vi "Header pkyk.vi"(8 "error in (no error)":errorcluster, 11 "New PKYK":T1) -> (0 "error out":errorcluster, 2 "MC No?":i32, 3 "PKYK":picture)   [LabVIEW 2020]
uses:
  MS SQL/MS_Global.vi
  Controls/Msg_Type.ctl
  Controls/Poka_Status.ctl
  Controls/PKYK_Status.ctl
  Controls/PKYK_Barcode_Status.ctl
  Controls/PKYK_qData.ctl
panel:
  # "Required\nResult"
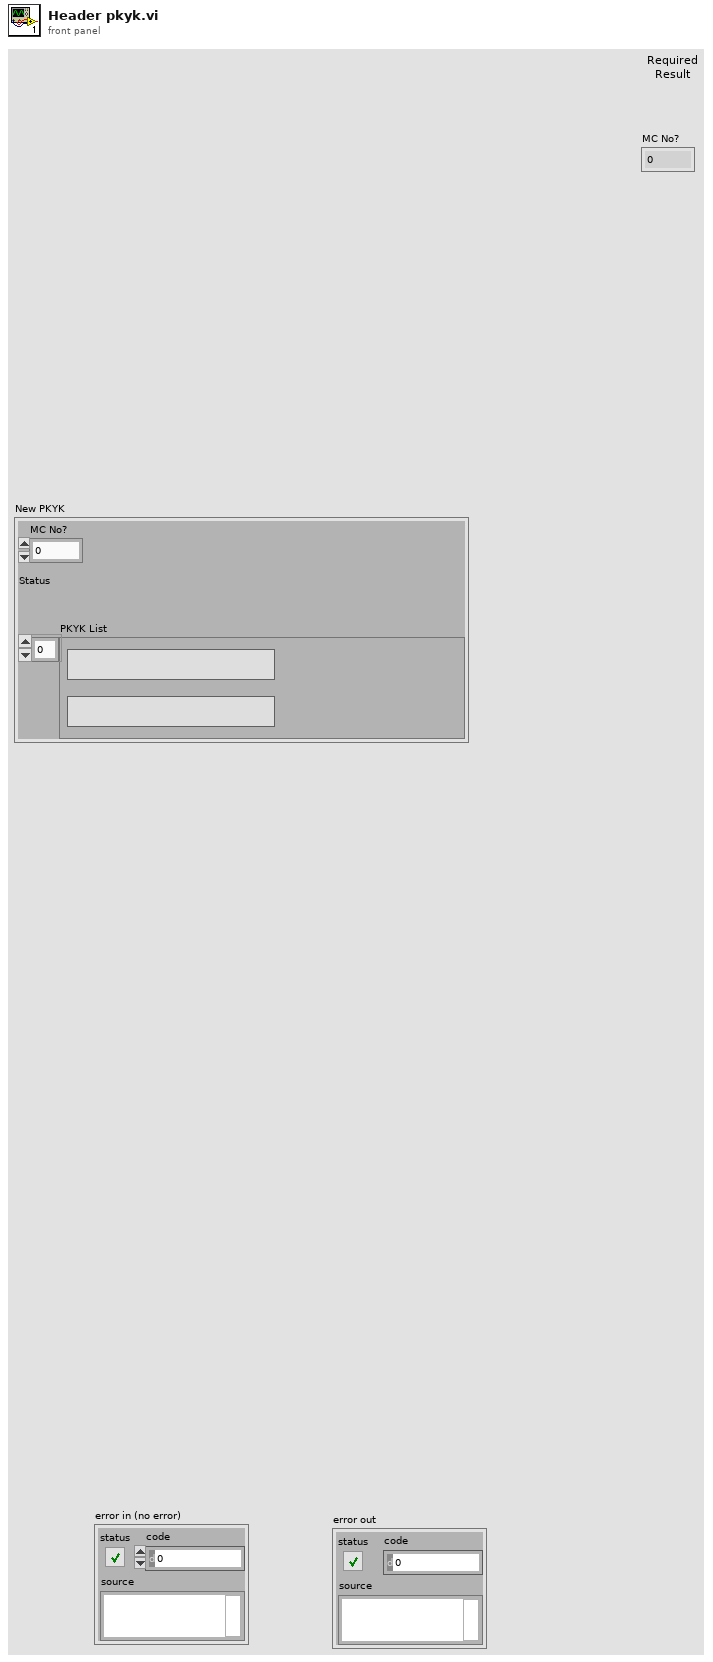
[diagram p1: front panel]
types:
  T1 = typedef "PKYK_qData.ctl" = cluster{"MC No?":i32, "Status":T2, "PKYK List":T3[]}
  T2 = typedef "Poka_Status.ctl" = u16
  T3 = typedef "PKYK_Barcode_Status.ctl" = cluster{"RFID Written Last":string, "Result":T4, "Exp. Result":T4}
  T4 = typedef "PKYK_Status.ctl" = u16
  T5 = typedef "Msg_Type.ctl" = enum16{"Normal", "Pass", "Fail", "Fault", "User", "Bypass", "Fail Save"}
  T6 = cluster{"left":i16, "top":i16, "right":i16, "bottom":i16}
  T7 = cluster{"Font Name:":string, "Size":i16, "Strikeout?":bool, "Italic?":bool, "Underline?":bool, "Outline?":bool, "Shadow?":bool, "Bold?":bool}
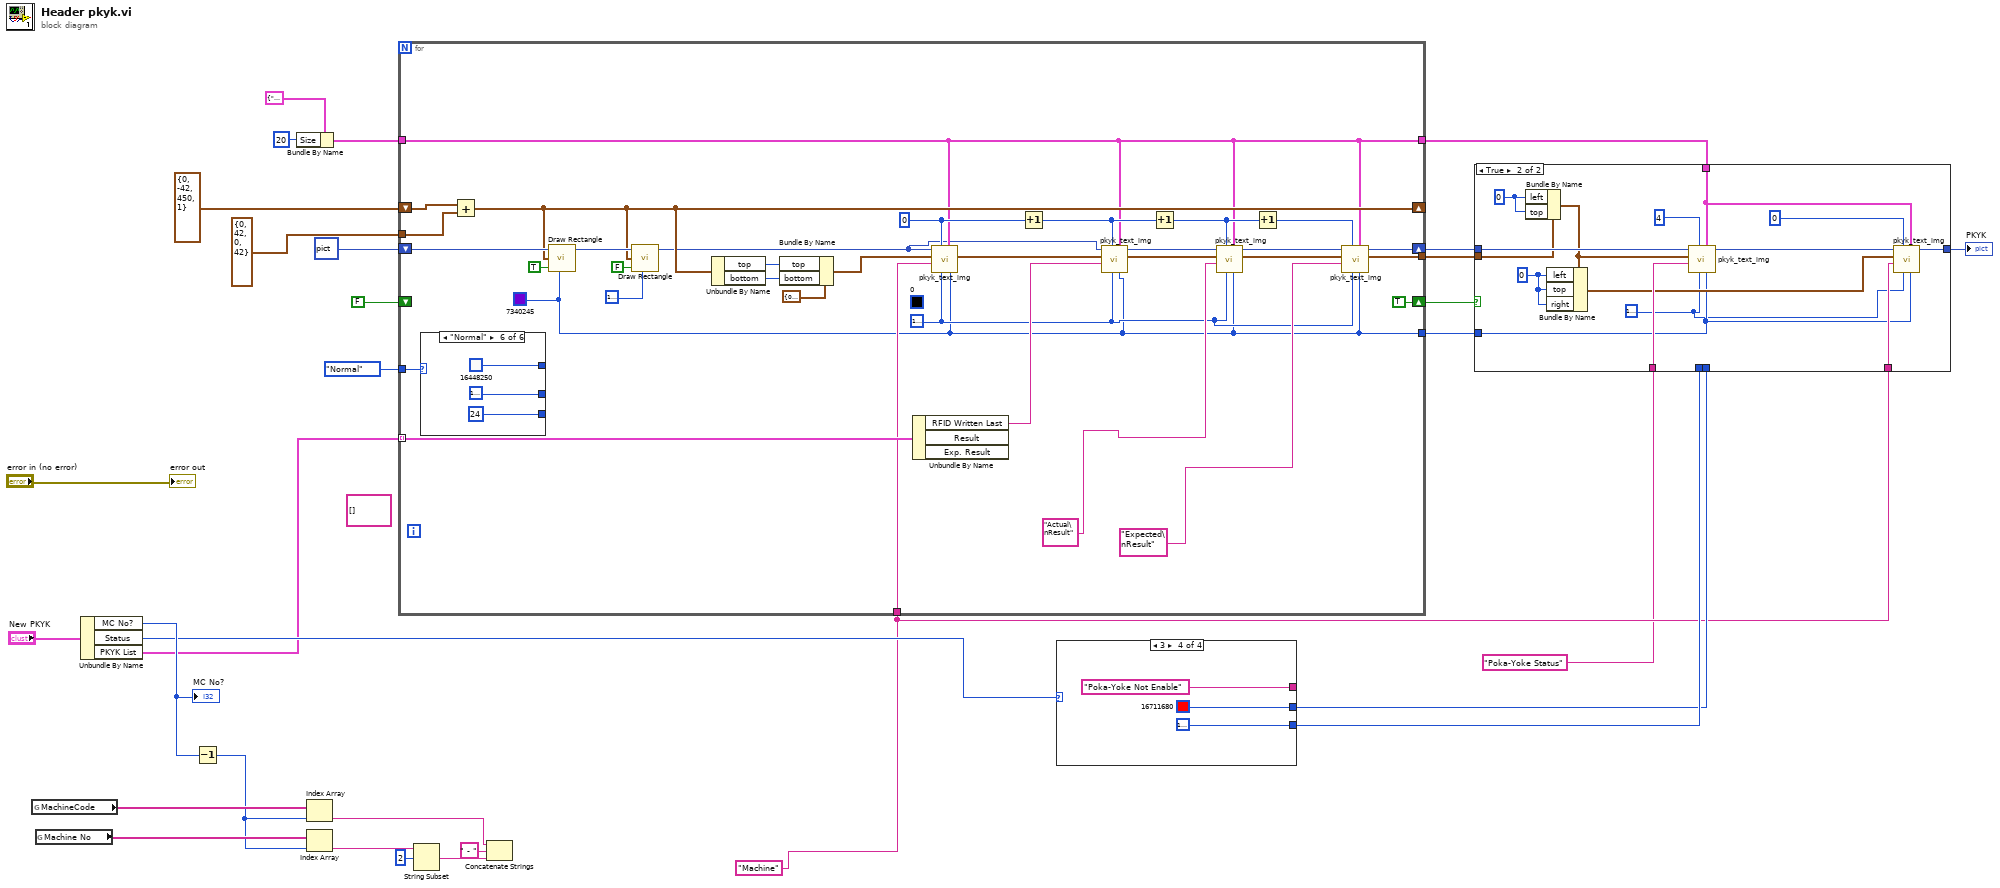
[diagram p0: block diagram]
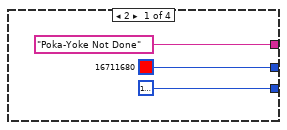
[diagram p3: hidden frame]
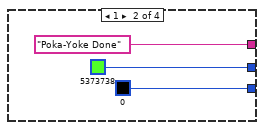
[diagram p4: hidden frame]
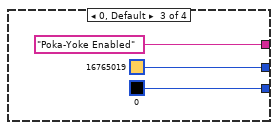
[diagram p5: hidden frame]
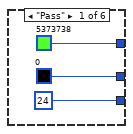
[diagram p6: hidden frame]
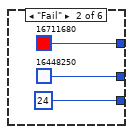
[diagram p7: hidden frame]
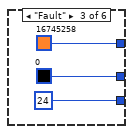
[diagram p8: hidden frame]
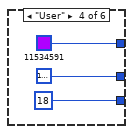
[diagram p9: hidden frame]
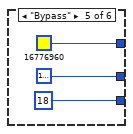
[diagram p10: hidden frame]
diagram:
  w3 = "Machine" ("concatenated string")
  (unwired) string[][] []
  n1 = global read "MS_Global.vi" "MachineCode"() -> (w30:string[])
  n2 = global read "MS_Global.vi" "Machine No"() -> (w29:string[])
  n3 = Unbundle By Name("New PKYK") -> ("MC No?"=w8:i32, "Status"=w7:T2, "PKYK List"=w6:T3[])
  "MC No?" <- w8
  n4 = Decrement(x=w8) -> (x-1=w10:i32)
  n5 = Bundle By Name(cluster=T7 {"Font Name:"="Segoe UI Semibold", "Size"=18, "Strikeout?"=FALSE, "Italic?"=FALSE, "Underline?"=FALSE, "Outline?"=FALSE, "Shadow?"=FALSE, "Bold?"=FALSE} ("[user-specified font]"), "Size"=i16 20) -> (w23:T7)
  n6 = Index Array(array=w30, index=w10) -> (element=w21:string)
  n7 = Index Array(array=w29, index=w10) -> (element=w27:string)
  n8 = for {
    tunnel: Msg_Type."Normal" ("Msg Type") -> [w61]
    tunnel: w23 -> [w38]
    tunnel: w3 -> [w56]
    tunnel: w6 -> [w60] mode=indexing
    shift-right: [w49] -> w14
    shift-left: picture data[5B] ("picture") -> [w59]
    shift-right: [w47] -> _
    shift-left: T6 {"left"=0, "top"=-42, "right"=450, "bottom"=1} ("output cluster") -> [w58]
    tunnel: T6 {"left"=0, "top"=42, "right"=0, "bottom"=42} ("output cluster") -> [w57]
    tunnel: [w39] -> w13
    tunnel: [w38] -> w12
    shift-right: [TRUE ("fill?(F)")] -> w4
    shift-left: FALSE ("fill?(F)") -> [_]
    tunnel: [w32] -> w2
    w32 = u32 7340245 ("color(black)")
    w43 = i16 0 ("Column")
    w33 = u32 16777226 ("color(black)")
    (unwired) u32 0 ("color(black)")
    n9 = case shown="\"Normal\"" w61 {
      tunnel: [u32 5373738 ("color(black)") u32 16711680 ("color(black)") u32 16745258 ("color(black)") u32 11534591 ("color(black)") u32 16776960 ("color(black)") u32 16448250 ("color(black)")] -> _
      tunnel: [u32 0 ("color(black)") u32 16448250 ("color(black)") u32 0 ("color(black)") u32 16777226 ("color(black)") u32 16777222 ("color(black)") u32 16777222 ("color(black)")] -> _
      tunnel: [i16 24 ("Size") i16 24 ("Size") i16 24 ("Size") i16 18 ("Size") i16 18 ("Size") i16 24 ("Size")] -> _
      frame "Pass" {
      }
      frame "Fail" {
      }
      frame "Fault" {
      }
      frame "User" {
      }
      frame "Bypass" {
      }
      frame "Normal" {
      }
    }
    n10 = Add(x=w58, y=w57) -> (x+y=w47:T6)
    n11 = call <vilib>:"Draw Rectangle.vi"("picture"=w59, "rect"=w47, "fill?(F)"=TRUE, "color(black)"=w32) -> ("new picture"=w63:picture)  [unwired: 5 in]
    n12 = call <vilib>:"Draw Rectangle.vi"("picture"=w63, "rect"=w47, "fill?(F)"=FALSE, "color(black)"=u32 16777226) -> ("new picture"=w37:picture)  [unwired: 5 in]
    n13 = Unbundle By Name(w47) -> ("top"=w46:i16, "bottom"=w45:i16)
    n14 = Bundle By Name(cluster=T6 {"left"=0, "top"=0, "right"=0, "bottom"=0} ("output cluster"), "top"=w46, "bottom"=w45) -> (w44:T6)
    n15 = Unbundle By Name(w60) -> ("RFID Written Last"=w54:string)  [unwired: 2 out]
    n16 = call "pkyk_text_img.vi"("Fill Color"=w32, "[user-specified font]"=w38, "Text Color"=w33, "Column"=w43, "Text"=w56, "Orgin In"=w44, "new picture in"=w37) -> ("Orgin Out"=w55:T6)  [unwired: 3 in, 1 out]
    n17 = Increment(x=w43) -> (x+1=w42:i16)
    n18 = call "pkyk_text_img.vi"("Fill Color"=w32, "[user-specified font]"=w38, "Text Color"=w33, "Column"=w42, "Text"=w54, "Orgin In"=w55, "new picture in"=w37) -> ("Orgin Out"=w52:T6, "new picture out"=w53:picture)  [unwired: 3 in]
    n19 = Increment(x=w42) -> (x+1=w41:i16)
    n20 = call "pkyk_text_img.vi"("Fill Color"=w32, "[user-specified font]"=w38, "Text Color"=w33, "Column"=w41, "Text"="Actual\nResult" ("RFID Written Last"), "Orgin In"=w52, "new picture in"=w53) -> ("Orgin Out"=w51:T6, "new picture out"=w50:picture)  [unwired: 3 in]
    n21 = Increment(x=w41) -> (x+1=w40:i16)
    n22 = call "pkyk_text_img.vi"("Fill Color"=w32, "[user-specified font]"=w38, "Text Color"=w33, "Column"=w40, "Text"="Expected\nResult" ("RFID Written Last"), "Orgin In"=w51, "new picture in"=w50) -> ("Orgin Out"=w39:T6, "new picture out"=w49:picture)  [unwired: 3 in]
  }
  n23 = String Subset(string=w27, offset (0)=2) -> (substring=w20:string)  [unwired: 1 in]
  n24 = Concatenate Strings(w21, " - " ("string"), w20) -> ()  [unwired: 1 out]
  n25 = case shown="3" w7 {
    tunnel: ["Poka-Yoke Not Done" ("Text") "Poka-Yoke Done" ("Text") "Poka-Yoke Enabled" ("Text") "Poka-Yoke Not Enable" ("Text")] -> _
    tunnel: [u32 16777226 ("color(black)") u32 0 ("color(black)") u32 0 ("color(black)") u32 16777226 ("color(black)")] -> w16
    tunnel: [u32 16711680 ("color(black)") u32 5373738 ("color(black)") u32 16765019 ("color(black)") u32 16711680 ("color(black)")] -> w15
    frame 2 {
    }
    frame 1 {
    }
    frame 0, Default {
    }
    frame 3 {
    }
  }
  n26 = case shown="True" w4 {
    tunnel: "Poka-Yoke Status" ("Text") -> [_ w111]
    tunnel: w16 -> [_ _]
    tunnel: w15 -> [_ _]
    tunnel: w14 -> [w96 w109]
    tunnel: w13 -> [_ w108]
    tunnel: w12 -> [_ w105]
    tunnel: [w96 w100] -> w11
    tunnel: w3 -> [_ w99]
    tunnel: w2 -> [_ w98]
    frame False {
    }
    frame True {
      w97 = u32 16777226 ("color(black)")
      w103 = i16 0 ("left")
      w107 = i16 0 ("left")
      n27 = Bundle By Name(cluster=w108, "left"=w107, "top"=w107) -> (w104:T6)
      n28 = Bundle By Name(cluster=w104, "left"=w103, "top"=w103, "right"=w103) -> (w102:T6)
      n29 = call "pkyk_text_img.vi"("Fill Color"=w98, "[user-specified font]"=w105, "Text Color"=w97, "Column"=i16 4, "Text"=w111, "Orgin In"=w104, "new picture in"=w109) -> ("new picture out"=w101:picture)  [unwired: 3 in, 1 out]
      n30 = call "pkyk_text_img.vi"("Fill Color"=w98, "[user-specified font]"=w105, "Text Color"=w97, "Column"=i16 0, "Text"=w99, "Orgin In"=w102, "new picture in"=w101) -> ("new picture out"=w100:picture)  [unwired: 3 in, 1 out]
    }
  }
  "PKYK" <- w11
  "error out" <- "error in (no error)"
